vi "API_DB.FindFirstSlot.vi"(6 "Timeout (ms)":u32, 7 "Wait (F)":bool, 8 "error in (no error)":errorcluster, 11 "DLP2 in":refnum<class "DLP2.lvclass">) -> (0 "error out":errorcluster, 2 "Slot":string, 3 "DLP2 out":refnum<class "DLP2.lvclass">)   [LabVIEW 2022 SP3, in "DLP2.lvclass"]
doc: "Developed by Kevin Thompson\nkevin@thompsonengineering.net\n\nCopyright 2018\nThompson Engineering, LLC"
uses:
  DLP2.lvclass
  DataTypes/AsynCmd_Temp01--enum.ctl
  DLP2.lvclass/DLP2.ctl
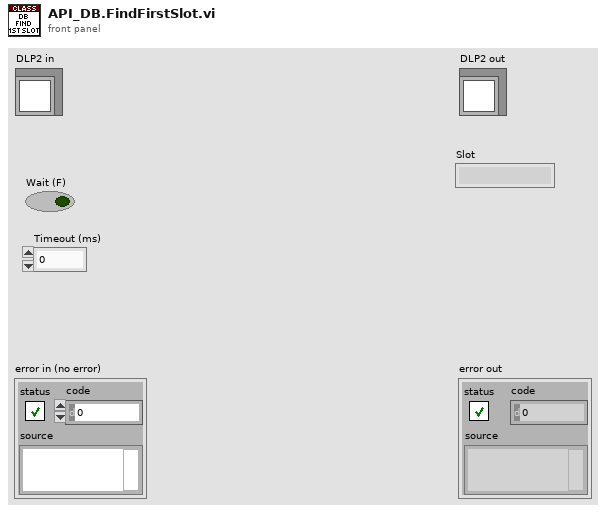
[diagram p1: front panel]
types:
  T1 = typedef "DLP2.lvclass/AsynCmd_Temp01--enum.ctl" = enum16{"DB.DeleteRecord", "DB.UpdateRecord", "DB.InsertRecord", "DB.SelectRecord", "DB.ExecuteSQLCommand", "DB.FindFirstSlot", "DB.GenericSQLQuery"}
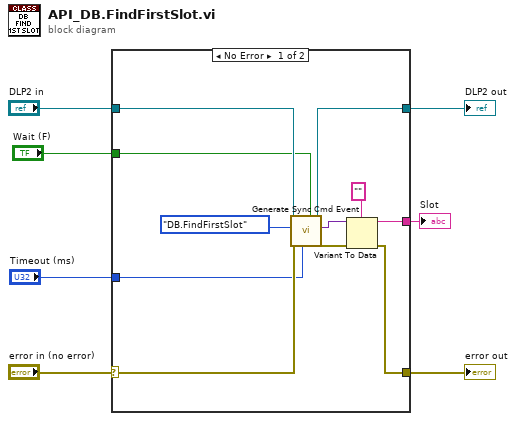
[diagram p0: block diagram]
diagram:
  n1 = case shown="No Error" "error in (no error)" {
    selector: "error in (no error)" -> [w16 w20]
    tunnel: [w11 w20] -> w6
    tunnel: [w17 w19] -> w4
    tunnel: "DLP2 in" -> [w18 w19]
    tunnel: [w13 _] -> w1
    tunnel: "Wait (F)" -> [w10 _]
    tunnel: "Timeout (ms)" -> [w9 _]
    frame No Error {
      n2 = call "Generate Sync Cmd Event.vi"("Wait (F)"=w10, "Timeout (ms)"=w9, "error in (no error)"=w16, "AsyncCmd"=AsynCmd_Temp01--enum."DB.FindFirstSlot", "DLP2 in"=w18) -> ("error out"=w12:errorcluster, "Return Value"=w14:variant, "DLP2 out"=w17:refnum<class "DLP2.lvclass">)  [unwired: 4 in]
      n3 = Variant To Data(error in=w12, type="", Variant=w14) -> (data=w13:string, error out=w11:errorcluster)
    }
    frame Error {
    }
  }
  "error out" <- w6
  "DLP2 out" <- w4
  "Slot" <- w1
